vi "Event--Shortcut Menu Selection.vi"(8 "error in":errorcluster, 10 "ItemPath":string, 11 "Selector in":refnum<class "Selector.lvclass">) -> (0 "error out":errorcluster, 2 "Selection":string, 3 "Selector out":refnum<class "Selector.lvclass">)   [LabVIEW 2019, in "Selector.lvclass"]
uses:
  Selector.lvclass
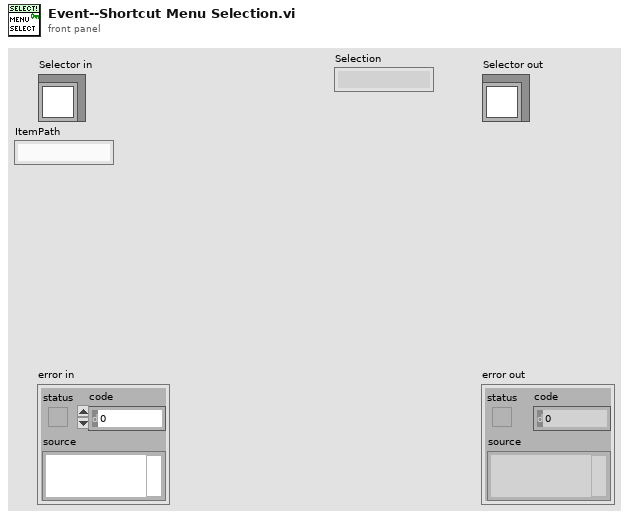
[diagram p1: front panel]
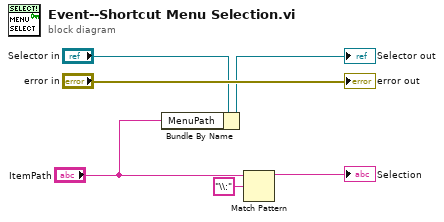
[diagram p0: block diagram]
diagram:
  n1 = Bundle By Name(cluster="Selector in", "MenuPath"="ItemPath") -> (→"Selector out":refnum<class "Selector.lvclass">)
  n2 = Match Pattern(string="ItemPath", regular expression="\\:") -> (before substring=→"Selection":string)  [unwired: 1 in, 3 out]
  "error out" <- "error in"
